vi "Read Measurement Data (Unit 1Chan).vi"(0 "VISA resource name":refnum<visa-resource-name>, 5 "Channel (1)":string="0001", 11 "error in (no error)":errorcluster) -> (4 "VISA resource name out":refnum<visa-resource-name>, 6 "Channel":string, 10 "Data Status":i32(ring) items=["Normal", "Differential Input", "Skip"], 13 "Decimal Position":i32 max=4 step=1, 14 "Unit":string, 15 "error out":errorcluster)   [LabVIEW 2020, in "Yokogawa GX Series.lvlib"]
doc: "This VI reads the channel number, data status, decimal position, and unit."
uses:
  <instrlib>/Yokogawa GX Series/Yokogawa GX Series.lvlib
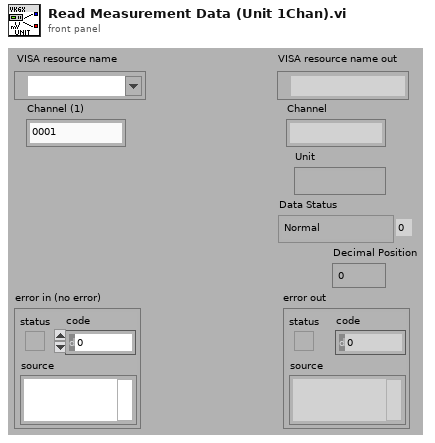
[diagram p1: front panel]
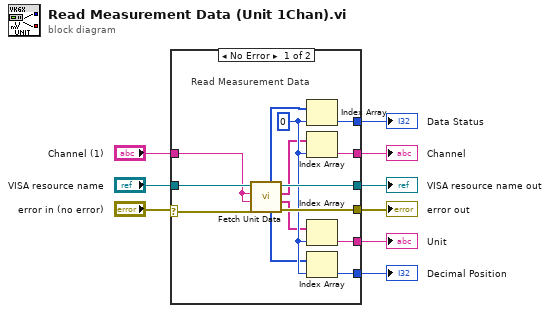
[diagram p0: block diagram]
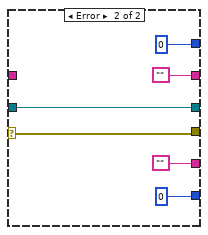
[diagram p2: hidden frame]
diagram:
  n1 = case shown="No Error" "error in (no error)" {
    selector: "error in (no error)" -> [w14 w28]
    tunnel: [w23 w29] -> w9
    tunnel: [w22 w28] -> w8
    tunnel: [w21 ""] -> w7
    tunnel: [w20 0] -> w6
    tunnel: [w19 0] -> w5
    tunnel: [w18 ""] -> w4
    tunnel: "VISA resource name" -> [w16 w29]
    tunnel: "Channel (1)" -> [w15 _]
    frame No Error {
      w17 = 0
      # "Read Measurement Data"
      n2 = call <instrlib>:"Fetch Unit Data.vi"("error in (no error)"=w14, "End Channel (1)"=w15, "Start Channel (1)"=w15, "VISA resource name"=w16) -> ("error out"=w22:errorcluster, "Unit"=w11:string[], "Channel"=w12:string[], "VISA resource name out"=w23:refnum<visa-resource-name>, "Decimal Position"=w10:i32[], "Data Status"=w13:i32[])  [unwired: 2 out]
      n3 = Index Array(array=w13, index=w17) -> (element=w20:i32)
      n4 = Index Array(array=w12, index=w17) -> (element=w21:string)
      n5 = Index Array(array=w11, index=w17) -> (element=w18:string)
      n6 = Index Array(array=w10, index=w17) -> (element=w19:i32)
    }
    frame Error {
    }
  }
  "error out" <- w8
  "VISA resource name out" <- w9
  "Unit" <- w4
  "Data Status" <- w6
  "Channel" <- w7
  "Decimal Position" <- w5
